vi "EnergyRangeToBragg.vi"(9 "FinalEnergy":dbl, 10 "InitalEnergy":dbl, 11 "EnergyStep":dbl) -> (3 "BraggArray":dbl[](array[numeric]))   [LabVIEW 2013]
panel:
  in  "E0":dbl=8300.0
  # "Angle in degrees"
  # "Back SkaTer energy"
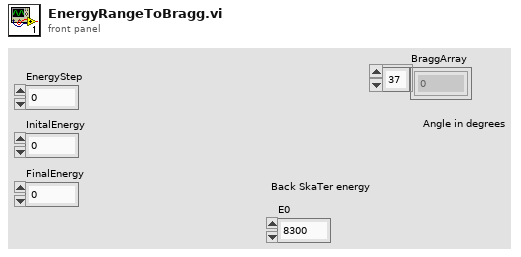
[diagram p1: front panel]
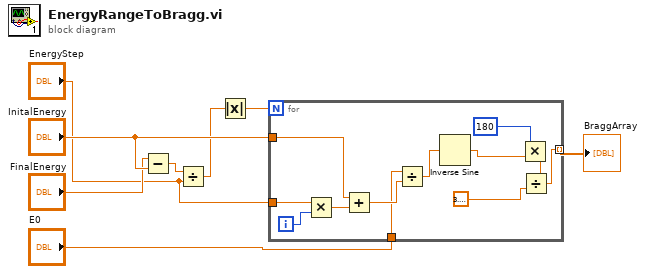
[diagram p0: block diagram]
diagram:
  n1 = Subtract(x="FinalEnergy", y="InitalEnergy") -> (x-y=w6:dbl)
  n2 = Divide(x=w6, y="EnergyStep") -> (x/y=w2:dbl)
  n3 = Absolute Value(x=w2) -> (abs(x)=w3:dbl)
  n4 = for {
    N: w3 -> [_]
    tunnel: "InitalEnergy" -> [w18]
    tunnel: [w12] -> w4 mode=indexing
    tunnel: "E0" -> [w16]
    tunnel: "EnergyStep" -> [w9]
    i -> [w20]
    n5 = Multiply(x=w9, y=w20) -> (x*y=w19:dbl)
    n6 = Add(x=w18, y=w19) -> (x+y=w17:dbl)
    n7 = Divide(x=w16, y=w17) -> (x/y=w15:dbl)
    n8 = Inverse Sine(1:w15) -> (0:w14:dbl)
    n9 = Multiply(x=180, y=w14) -> (x*y=w13:dbl)
    n10 = Divide(x=w13, y=3.141592653589793) -> (x/y=w12:dbl)
  }
  "BraggArray" <- w4
